vi "Frict.vi"(8 "FrictH":dbl, 9 "hldU":dbl, 10 "FrictD":dbl, 11 "dirU":dbl) -> (0 "hldU":dbl, 2 "dirU":dbl)   [LabVIEW 2013]
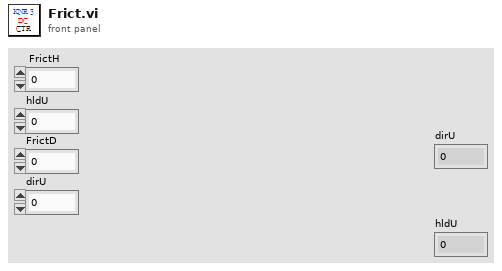
[diagram p1: front panel]
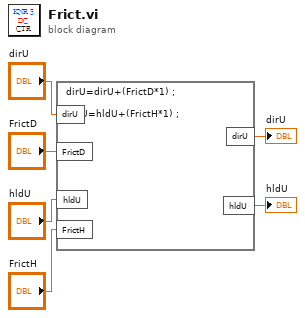
[diagram p0: block diagram]
diagram:
  n1 = formula code="dirU=dirU+(FrictD*1) ; \n\nhldU=hldU+(FrictH*1) ;"("dirU"="dirU", "FrictD"="FrictD", "hldU"="hldU", "FrictH"="FrictH") -> ("dirU"=→"dirU":dbl, "hldU"=→"hldU":dbl)
